vi "FGVWaveformShape.vi"(6 "Framing up? (down: f) In":bool=TRUE, 7 "Enum":T2, 8 "error in":errorcluster, 9 "Waveform Shape Slow In":dbl[](array[numeric]), 10 "Waveform Shape Fast In":dbl[](array[numeric])) -> (0 "error out":errorcluster, 1 "Waveform Shape Slow Out":dbl[](array[numeric]), 2 "Waveform Shape Fast Out":dbl[](array[numeric]), 3 "WaveformInit":T1, 4 "Framing up? (down: f) out":bool=TRUE)   [LabVIEW 2016]
uses:
  controls/Enum.ctl
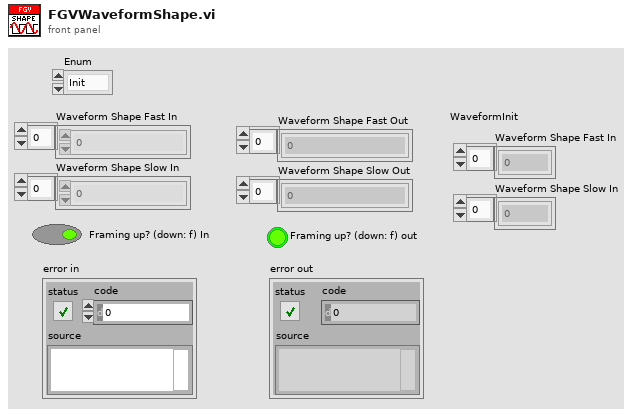
[diagram p1: front panel]
types:
  T1 = cluster{"Waveform Shape Fast In":dbl[], "Waveform Shape Slow In":dbl[]}
  T2 = typedef "Enum.ctl" = enum16{"Init", "Read", "Write"}
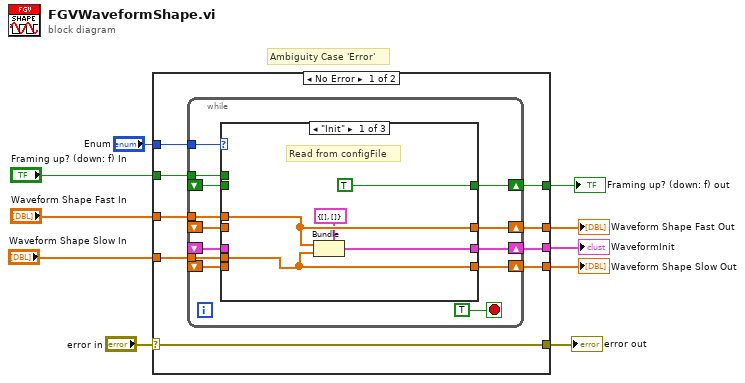
[diagram p0: block diagram]
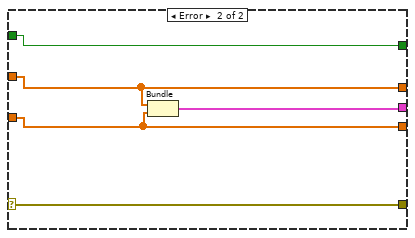
[diagram p4: hidden frame]
diagram:
  # "Ambiguity Case 'Error'"
  n1 = case shown="No Error" "error in" {
    selector: "error in" -> [w18 w50]
    tunnel: "Enum" -> [w19 _]
    tunnel: [w18 w50] -> w9
    tunnel: "Waveform Shape Slow In" -> [w17 w46]
    tunnel: [w16 w46] -> w5
    tunnel: "Waveform Shape Fast In" -> [w15 w47]
    tunnel: [w14 w47] -> w4
    tunnel: "Framing up? (down: f) In" -> [w13 w49]
    tunnel: [w12 w49] -> w1
    tunnel: [w11 w48] -> w3
    frame No Error {
      n2 = while {
        tunnel: w19 -> [w31]
        tunnel: w17 -> [w30]
        shift-right: [w29] -> w16
        shift-left: _ -> [w28]
        tunnel: w15 -> [w27]
        shift-right: [w26] -> w14
        shift-left: _ -> [w25]
        tunnel: w13 -> [w24]
        shift-right: [w23] -> w12
        shift-left: _ -> [w22]
        shift-right: [w21] -> w11
        shift-left: _ -> [w20]
        stop <- TRUE stop-if-true
        n3 = case shown="\"Init\"" w31 {
          tunnel: w30 -> [w35 _ w45]
          tunnel: [w35 w41 w45] -> w29
          tunnel: w28 -> [_ w41 _]
          tunnel: w27 -> [w36 _ w44]
          tunnel: [w36 w40 w44] -> w26
          tunnel: w25 -> [_ w40 _]
          tunnel: w24 -> [_ _ w43]
          tunnel: [TRUE ("Framing up? (down: f)") w39 w43] -> w23
          tunnel: w22 -> [_ w39 _]
          tunnel: [w37 w38 w42] -> w21
          tunnel: w20 -> [_ w38 w42]
          frame "Init" {
            # "Read from configFile"
            n4 = Bundle(cluster=T1 {"Waveform Shape Fast In"=[], "Waveform Shape Slow In"=[]} ("output cluster"), "Waveform Shape Fast In"=w36, "Waveform Shape Slow In"=w35) -> (w37:T1)
          }
          frame "Read", Default {
          }
          frame "Write" {
          }
        }
      }
    }
    frame Error {
      n5 = Bundle("Waveform Shape Fast In"=w47, "Waveform Shape Slow In"=w46) -> (w48:T1)  [unwired: 1 in]
    }
  }
  "error out" <- w9
  "Waveform Shape Slow Out" <- w5
  "Waveform Shape Fast Out" <- w4
  "WaveformInit" <- w3
  "Framing up? (down: f) out" <- w1
